vi "Connect.vi"(8 "error in (no error)":errorcluster, 9 "timeout":i32=-1, 11 "Network Stream Initiator in":refnum<class "Network Stream Initiator.lvclass">=refnum) -> (0 "error out":errorcluster, 3 "Network Stream Initiator out":refnum<class "Network Stream Initiator.lvclass">)   [LabVIEW 2023, in "Network Stream Initiator.lvclass"]
doc: "This method initiates a connection between a Network Stream Initiator/Listener pair."
uses:
  Network Stream Initiator.lvclass
  Network Stream/Network Stream.lvclass
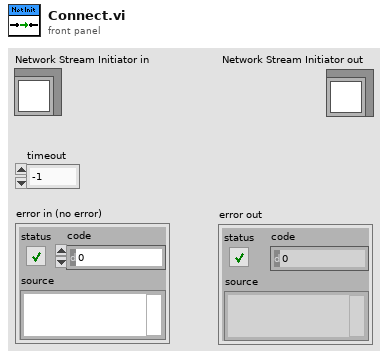
[diagram p1: front panel]
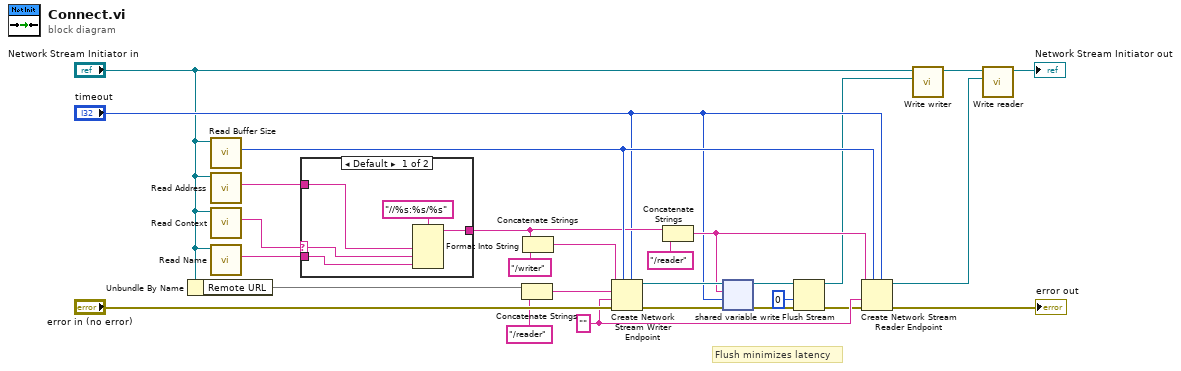
[diagram p0: block diagram]
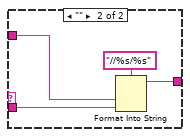
[diagram p2: hidden frame]
diagram:
  w21 = ""
  # "Flush minimizes latency"
  n1 = Unbundle By Name("Network Stream Initiator in") -> ("Remote URL"=w26)
  n2 = call "Read Buffer Size.vi"("Network Stream in"="Network Stream Initiator in") -> ("Buffer Size"=w22:i32)  [unwired: 10 in]
  n3 = call "Read Address.vi"("Network Stream in"="Network Stream Initiator in") -> ("Address"=w1:string)  [unwired: 10 in]
  n4 = call "Read Context.vi"("Network Stream in"="Network Stream Initiator in") -> ("Context"=w24:string)  [unwired: 10 in]
  n5 = call "Read Name.vi"("Network Stream in"="Network Stream Initiator in") -> ("Name"=w25:string)  [unwired: 10 in]
  n6 = case shown="Default" w24 {
    selector: w24 -> [w29 _]
    tunnel: [w31 w36] -> w15
    tunnel: w25 -> [w30 w34]
    tunnel: w1 -> [w28 w33]
    frame Default {
      n7 = Format Into String(format string="//%s:%s/%s", w28, w29, w30) -> (resulting string=w31:string)  [unwired: 2 in, 1 out]
    }
    frame "" {
      n8 = Format Into String(format string="//%s/%s", w33, w34) -> (resulting string=w36:string)  [unwired: 2 in, 1 out]
    }
  }
  n9 = Concatenate Strings(w26, "/reader" ("format string")) -> (w19:string)
  n10 = Concatenate Strings(w15, "/writer" ("format string")) -> (w17:string)
  n11 = Create Network Stream Writer Endpoint(5:"timeout", 7:w22, 8:"error in (no error)", 9:w21, 10:w19, 11:w17) -> (0:w14:errorcluster, 3:w13:refnum<k21>)  [unwired: 1 in]
  n12 = Concatenate Strings(w15, "/reader" ("format string")) -> (w12:string)
  n13 = shared-variable-write(w13, w14, w12, "timeout") -> (w4:refnum<k21>, w6:errorcluster)  [unwired: 1 out]
  n14 = Flush Stream(8:w6, 9:0 ("timeout in ms (-1)"), 11:w4) -> (0:w5:errorcluster, 3:w3:refnum<k21>)  [unwired: 1 in, 1 out]
  n15 = Create Network Stream Reader Endpoint(5:"timeout", 7:w22, 8:w5, 9:w21, 11:w12) -> (0:→"error out":errorcluster, 3:w10:refnum<k21>)  [unwired: 2 in]
  n16 = call "Write writer.vi"("writer"=w3, "Network Stream in"="Network Stream Initiator in") -> ("Network Stream out"=w9:refnum<class "Network Stream.lvclass">)  [unwired: 9 in]
  n17 = call "Write reader.vi"("reader"=w10, "Network Stream in"=w9) -> ("Network Stream out"=→"Network Stream Initiator out":refnum<class "Network Stream.lvclass">)  [unwired: 9 in]
